vi "200_RED TO BLUE.vi"   [LabVIEW 2019]
uses:
  Global Var.vi
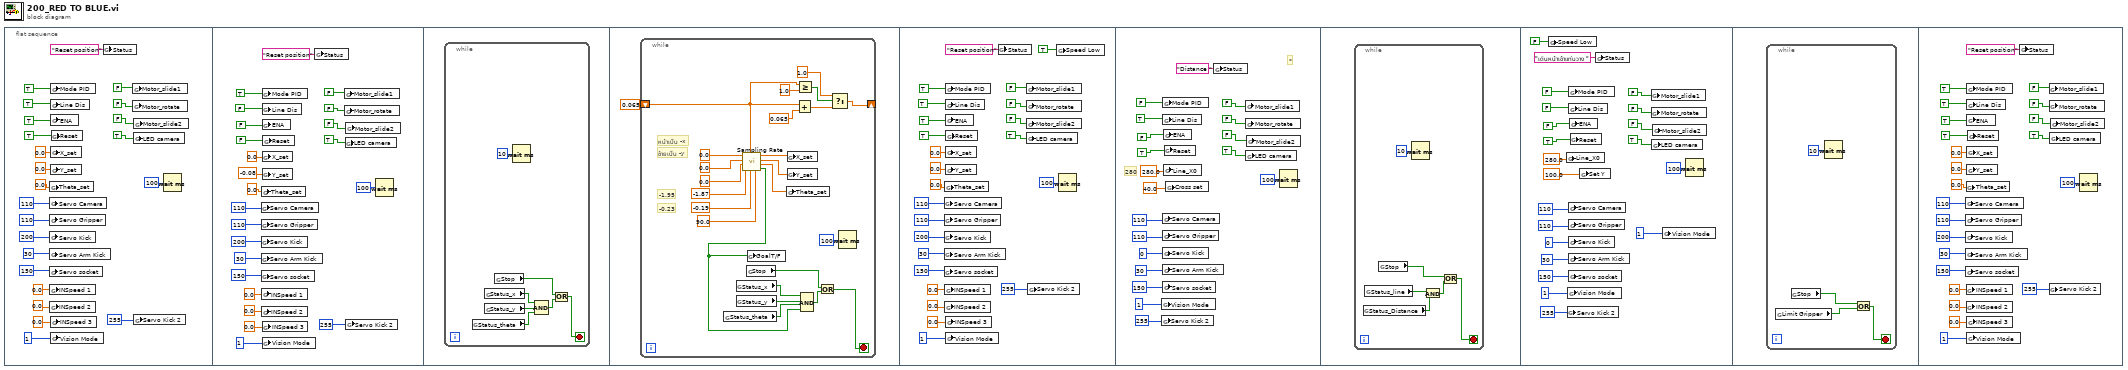
[diagram p0: block diagram]
diagram:
  n1 = flat-sequence {
    frame #0 {
      n2 = global write "Global Var.vi" "Servo Camera"(u8 110 ("Servo Camera")) -> ()
      n3 = global write "Global Var.vi" "Servo Gripper"(u8 110 ("Servo Camera")) -> ()
      n4 = global write "Global Var.vi" "Servo Kick"(u8 200 ("Servo Camera")) -> ()
      n5 = global write "Global Var.vi" "Servo Arm Kick"(u8 30 ("Servo Camera")) -> ()
      n6 = global write "Global Var.vi" "Servo socket"(u8 150 ("Servo Camera")) -> ()
      n7 = global write "Global Var.vi" "Theta_set"(0.0 ("Theta_set")) -> ()
      n8 = global write "Global Var.vi" "INSpeed 1"(0.0 ("X_set")) -> ()
      n9 = global write "Global Var.vi" "INSpeed 2"(0.0 ("Y_set")) -> ()
      n10 = global write "Global Var.vi" "Mode PID"(TRUE ("Mode PID")) -> ()
      n11 = global write "Global Var.vi" "Line Dis"(TRUE ("Mode PID")) -> ()
      n12 = global write "Global Var.vi" "ENA"(TRUE ("ENA")) -> ()
      n13 = global write "Global Var.vi" "X_set"(0.0 ("X_set")) -> ()
      n14 = global write "Global Var.vi" "Y_set"(0.0 ("Y_set")) -> ()
      n15 = global write "Global Var.vi" "INSpeed 3"(0.0 ("Theta_set")) -> ()
      n16 = global write "Global Var.vi" "Vision Mode"(i16 1 ("Vision Mode")) -> ()
      n17 = global write "Global Var.vi" "Reset"(TRUE ("ENA")) -> ()
      n18 = global write "Global Var.vi" "Status"("Reset position" ("Status")) -> ()
      n19 = global write "Global Var.vi" "Motor_slide1"(FALSE ("Mode PID")) -> ()
      n20 = global write "Global Var.vi" "Motor_rotate"(FALSE ("ENA")) -> ()
      n21 = global write "Global Var.vi" "LED camera"(TRUE ("LED camera")) -> ()
      n22 = global write "Global Var.vi" "Motor_slide2"(FALSE ("ENA")) -> ()
      n23 = global write "Global Var.vi" "Servo Kick 2"(u8 255 ("Servo Camera")) -> ()
      n24 = Wait (ms)(milliseconds to wait=u32 100) -> ()  [unwired: 1 out]
    }
    frame #1 {
      n25 = global write "Global Var.vi" "Servo Camera"(u8 110 ("Servo Camera")) -> ()
      n26 = global write "Global Var.vi" "Servo Gripper"(u8 110 ("Servo Camera")) -> ()
      n27 = global write "Global Var.vi" "Servo Kick"(u8 200 ("Servo Camera")) -> ()
      n28 = global write "Global Var.vi" "Servo Arm Kick"(u8 30 ("Servo Camera")) -> ()
      n29 = global write "Global Var.vi" "Servo socket"(u8 150 ("Servo Camera")) -> ()
      n30 = global write "Global Var.vi" "Theta_set"(0.0 ("Theta_set")) -> ()
      n31 = global write "Global Var.vi" "INSpeed 1"(0.0 ("X_set")) -> ()
      n32 = global write "Global Var.vi" "INSpeed 2"(0.0 ("Y_set")) -> ()
      n33 = global write "Global Var.vi" "Mode PID"(TRUE ("Mode PID")) -> ()
      n34 = global write "Global Var.vi" "Line Dis"(FALSE ("Mode PID")) -> ()
      n35 = global write "Global Var.vi" "ENA"(FALSE ("ENA")) -> ()
      n36 = global write "Global Var.vi" "X_set"(0.0 ("X_set")) -> ()
      n37 = global write "Global Var.vi" "Y_set"(-0.08 ("Y_set")) -> ()
      n38 = global write "Global Var.vi" "INSpeed 3"(0.0 ("Theta_set")) -> ()
      n39 = global write "Global Var.vi" "Vision Mode"(i16 1 ("Vision Mode")) -> ()
      n40 = global write "Global Var.vi" "Reset"(FALSE ("ENA")) -> ()
      n41 = global write "Global Var.vi" "Status"("Reset position" ("Status")) -> ()
      n42 = global write "Global Var.vi" "Motor_slide1"(FALSE ("Mode PID")) -> ()
      n43 = global write "Global Var.vi" "Motor_rotate"(FALSE ("ENA")) -> ()
      n44 = global write "Global Var.vi" "LED camera"(TRUE ("LED camera")) -> ()
      n45 = global write "Global Var.vi" "Motor_slide2"(FALSE ("ENA")) -> ()
      n46 = global write "Global Var.vi" "Servo Kick 2"(u8 255 ("Servo Camera")) -> ()
      n47 = Wait (ms)(milliseconds to wait=u32 100) -> ()  [unwired: 1 out]
    }
    frame #2 {
      n48 = while {
        stop <- w49 stop-if-true
        n49 = global read "Global Var.vi" "Status_theta"() -> (w51:bool)
        n50 = global read "Global Var.vi" "Status_x"() -> (w52:bool)
        n51 = global read "Global Var.vi" "Status_y"() -> (w53:bool)
        n52 = global read "Global Var.vi" "Stop"() -> (w47:bool)
        n53 = Wait (ms)(milliseconds to wait=u32 10) -> ()  [unwired: 1 out]
        n54 = Compound Arithmetic op=AND(w52, w53, w51) -> (w48:bool)
        n55 = Or(x=w47, y=w48) -> (x .or. y?=w49:bool)
      }
    }
    frame #3 {
      n56 = while {
        shift-right: [w57] -> _
        shift-left: 0.065 -> [w55]
        stop <- w74 stop-if-true
        # "-0.23"
        # "-1.95"
        # "ซ้ายเป็น -y"
        # "หน้าเป็น -x"
        n57 = global read "Global Var.vi" "Status_theta"() -> (w76:bool)
        n58 = global read "Global Var.vi" "Status_x"() -> (w77:bool)
        n59 = global read "Global Var.vi" "Status_y"() -> (w78:bool)
        n60 = call "Sampling Rate.vi"("input a1"=90.0, "input y1"=-0.19, "T(0-1)"=w55, "input x1"=-1.87, "input a0"=0.0, "input y0"=0.0, "input x0"=0.0) -> ("GoalT/F"=w62:bool, "a_output"=w69:dbl, "y_output"=w70:dbl, "x_output"=w71:dbl)  [unwired: 1 in]
        n61 = global read "Global Var.vi" "Stop"() -> (w72:bool)
        n62 = global write "Global Var.vi" "GoalT/F"(w62) -> ()
        n63 = global write "Global Var.vi" "Theta_set"(w69) -> ()
        n64 = global write "Global Var.vi" "X_set"(w71) -> ()
        n65 = global write "Global Var.vi" "Y_set"(w70) -> ()
        n66 = Add(x=w55, y=0.065) -> (x+y=w60:dbl)
        n67 = Greater Or Equal?(x=w55, y=1.0) -> (x >= y?=w59:bool)
        n68 = Compound Arithmetic op=AND(w77, w78, w76, w62) -> (w73:bool)
        n69 = Or(x=w72, y=w73) -> (x .or. y?=w74:bool)
        n70 = Select(t=1.0, s=w59, f=w60) -> (s? t:f=w57:dbl)
        n71 = Wait (ms)(milliseconds to wait=u32 100) -> ()  [unwired: 1 out]
      }
    }
    frame #4 {
      n72 = global write "Global Var.vi" "Servo Camera"(u8 110 ("Servo Camera")) -> ()
      n73 = global write "Global Var.vi" "Servo Gripper"(u8 110 ("Servo Camera")) -> ()
      n74 = global write "Global Var.vi" "Servo Kick"(u8 200 ("Servo Camera")) -> ()
      n75 = global write "Global Var.vi" "Servo Arm Kick"(u8 30 ("Servo Camera")) -> ()
      n76 = global write "Global Var.vi" "Servo socket"(u8 150 ("Servo Camera")) -> ()
      n77 = global write "Global Var.vi" "Theta_set"(0.0 ("Theta_set")) -> ()
      n78 = global write "Global Var.vi" "INSpeed 1"(0.0 ("X_set")) -> ()
      n79 = global write "Global Var.vi" "INSpeed 2"(0.0 ("Y_set")) -> ()
      n80 = global write "Global Var.vi" "Mode PID"(TRUE ("Mode PID")) -> ()
      n81 = global write "Global Var.vi" "Line Dis"(TRUE ("Mode PID")) -> ()
      n82 = global write "Global Var.vi" "ENA"(TRUE ("ENA")) -> ()
      n83 = global write "Global Var.vi" "X_set"(0.0 ("X_set")) -> ()
      n84 = global write "Global Var.vi" "Y_set"(0.0 ("Y_set")) -> ()
      n85 = global write "Global Var.vi" "INSpeed 3"(0.0 ("Theta_set")) -> ()
      n86 = global write "Global Var.vi" "Vision Mode"(i16 1 ("Vision Mode")) -> ()
      n87 = global write "Global Var.vi" "Reset"(TRUE ("ENA")) -> ()
      n88 = global write "Global Var.vi" "Status"("Reset position" ("Status")) -> ()
      n89 = global write "Global Var.vi" "Motor_slide1"(FALSE ("Mode PID")) -> ()
      n90 = global write "Global Var.vi" "Motor_rotate"(FALSE ("ENA")) -> ()
      n91 = global write "Global Var.vi" "Motor_slide2"(FALSE ("ENA")) -> ()
      n92 = global write "Global Var.vi" "LED camera"(TRUE ("LED camera")) -> ()
      n93 = global write "Global Var.vi" "Servo Kick 2"(u8 255 ("Servo Camera")) -> ()
      n94 = global write "Global Var.vi" "Speed Low"(TRUE ("LED camera")) -> ()
      n95 = Wait (ms)(milliseconds to wait=u32 100) -> ()  [unwired: 1 out]
    }
    frame #5 {
      # "280"
      # "*"
      n96 = global write "Global Var.vi" "Vision Mode"(i16 1 ("Vision Mode")) -> ()
      n97 = global write "Global Var.vi" "Servo Kick 2"(u8 255 ("Servo Camera")) -> ()
      n98 = global write "Global Var.vi" "Servo Camera"(u8 110 ("Servo Camera")) -> ()
      n99 = global write "Global Var.vi" "Servo Gripper"(u8 110 ("Servo Camera")) -> ()
      n100 = global write "Global Var.vi" "Servo Kick"(u8 0 ("Servo Camera")) -> ()
      n101 = global write "Global Var.vi" "Servo Arm Kick"(u8 30 ("Servo Camera")) -> ()
      n102 = global write "Global Var.vi" "Servo socket"(u8 150 ("Servo Camera")) -> ()
      n103 = global write "Global Var.vi" "Mode PID"(FALSE ("Mode PID")) -> ()
      n104 = global write "Global Var.vi" "Line Dis"(TRUE ("Mode PID")) -> ()
      n105 = global write "Global Var.vi" "ENA"(FALSE ("ENA")) -> ()
      n106 = global write "Global Var.vi" "Line_X0"(280.0 ("Y_set")) -> ()
      n107 = global write "Global Var.vi" "Reset"(TRUE ("ENA")) -> ()
      n108 = global write "Global Var.vi" "Cross set"(40.0 ("Y_set")) -> ()
      n109 = global write "Global Var.vi" "Status"("Distance " ("Status")) -> ()
      n110 = global write "Global Var.vi" "Motor_slide1"(FALSE ("Mode PID")) -> ()
      n111 = global write "Global Var.vi" "Motor_rotate"(FALSE ("ENA")) -> ()
      n112 = global write "Global Var.vi" "LED camera"(TRUE ("LED camera")) -> ()
      n113 = global write "Global Var.vi" "Motor_slide2"(FALSE ("ENA")) -> ()
      n114 = Wait (ms)(milliseconds to wait=u32 100) -> ()  [unwired: 1 out]
    }
    frame #6 {
      n115 = while {
        stop <- w126 stop-if-true
        n116 = global read "Global Var.vi" "Status_Distance"() -> (w122:bool)
        n117 = global read "Global Var.vi" "Status_line"() -> (w123:bool)
        n118 = global read "Global Var.vi" "Stop"() -> (w125:bool)
        n119 = Wait (ms)(milliseconds to wait=u32 10) -> ()  [unwired: 1 out]
        n120 = And(x=w123, y=w122) -> (x .and. y?=w124:bool)
        n121 = Or(x=w125, y=w124) -> (x .or. y?=w126:bool)
      }
    }
    frame #7 {
      n122 = global write "Global Var.vi" "Speed Low"(FALSE ("LED camera")) -> ()
      n123 = global write "Global Var.vi" "Line_X0"(280.0 ("Y_set")) -> ()
      n124 = global write "Global Var.vi" "Servo Kick 2"(u8 255 ("Servo Camera")) -> ()
      n125 = global write "Global Var.vi" "Vision Mode"(i16 1 ("Vision Mode")) -> ()
      n126 = global write "Global Var.vi" "Servo Camera"(u8 110 ("Servo Camera")) -> ()
      n127 = global write "Global Var.vi" "Servo Gripper"(u8 110 ("Servo Camera")) -> ()
      n128 = global write "Global Var.vi" "Servo Kick"(u8 0 ("Servo Camera")) -> ()
      n129 = global write "Global Var.vi" "Servo Arm Kick"(u8 30 ("Servo Camera")) -> ()
      n130 = global write "Global Var.vi" "Servo socket"(u8 150 ("Servo Camera")) -> ()
      n131 = global write "Global Var.vi" "Mode PID"(FALSE ("Mode PID")) -> ()
      n132 = global write "Global Var.vi" "Line Dis"(FALSE ("Mode PID")) -> ()
      n133 = global write "Global Var.vi" "ENA"(FALSE ("ENA")) -> ()
      n134 = global write "Global Var.vi" "Reset"(TRUE ("ENA")) -> ()
      n135 = global write "Global Var.vi" "Set Y"(100.0 ("Y_set")) -> ()
      n136 = global write "Global Var.vi" "Status"("เดินหน้าเข้าแท่นวาง " ("Status")) -> ()
      n137 = global write "Global Var.vi" "Motor_slide1"(FALSE ("Mode PID")) -> ()
      n138 = global write "Global Var.vi" "Motor_rotate"(FALSE ("ENA")) -> ()
      n139 = global write "Global Var.vi" "LED camera"(TRUE ("LED camera")) -> ()
      n140 = global write "Global Var.vi" "Motor_slide2"(FALSE ("ENA")) -> ()
      n141 = global write "Global Var.vi" "Vision Mode"(i16 1 ("Vision Mode")) -> ()
      n142 = Wait (ms)(milliseconds to wait=u32 100) -> ()  [unwired: 1 out]
    }
    frame #8 {
      n143 = while {
        stop <- w151 stop-if-true
        n144 = global read "Global Var.vi" "Limit Gripper"() -> (w149:bool)
        n145 = global read "Global Var.vi" "Stop"() -> (w150:bool)
        n146 = Wait (ms)(milliseconds to wait=u32 10) -> ()  [unwired: 1 out]
        n147 = Or(x=w150, y=w149) -> (x .or. y?=w151:bool)
      }
    }
    frame #9 {
      n148 = global write "Global Var.vi" "Servo Camera"(u8 110 ("Servo Camera")) -> ()
      n149 = global write "Global Var.vi" "Servo Gripper"(u8 110 ("Servo Camera")) -> ()
      n150 = global write "Global Var.vi" "Servo Kick"(u8 200 ("Servo Camera")) -> ()
      n151 = global write "Global Var.vi" "Servo Arm Kick"(u8 30 ("Servo Camera")) -> ()
      n152 = global write "Global Var.vi" "Servo socket"(u8 150 ("Servo Camera")) -> ()
      n153 = global write "Global Var.vi" "Theta_set"(0.0 ("Theta_set")) -> ()
      n154 = global write "Global Var.vi" "INSpeed 1"(0.0 ("X_set")) -> ()
      n155 = global write "Global Var.vi" "INSpeed 2"(0.0 ("Y_set")) -> ()
      n156 = global write "Global Var.vi" "Mode PID"(TRUE ("Mode PID")) -> ()
      n157 = global write "Global Var.vi" "Line Dis"(TRUE ("Mode PID")) -> ()
      n158 = global write "Global Var.vi" "ENA"(TRUE ("ENA")) -> ()
      n159 = global write "Global Var.vi" "X_set"(0.0 ("X_set")) -> ()
      n160 = global write "Global Var.vi" "Y_set"(0.0 ("Y_set")) -> ()
      n161 = global write "Global Var.vi" "INSpeed 3"(0.0 ("Theta_set")) -> ()
      n162 = global write "Global Var.vi" "Vision Mode"(i16 1 ("Vision Mode")) -> ()
      n163 = global write "Global Var.vi" "Reset"(TRUE ("ENA")) -> ()
      n164 = global write "Global Var.vi" "Status"("Reset position" ("Status")) -> ()
      n165 = global write "Global Var.vi" "Motor_slide1"(FALSE ("Mode PID")) -> ()
      n166 = global write "Global Var.vi" "Motor_rotate"(FALSE ("ENA")) -> ()
      n167 = global write "Global Var.vi" "Servo Kick 2"(u8 255 ("Servo Camera")) -> ()
      n168 = global write "Global Var.vi" "LED camera"(TRUE ("LED camera")) -> ()
      n169 = global write "Global Var.vi" "Motor_slide2"(FALSE ("ENA")) -> ()
      n170 = Wait (ms)(milliseconds to wait=u32 100) -> ()  [unwired: 1 out]
    }
  }
